vi "CloseSession.vi"   [LabVIEW 2023]
uses:
  Open_device_2018.llb/Select_Instr.ctl
types:
  T1 = typedef "Select_Instr.ctl" = string
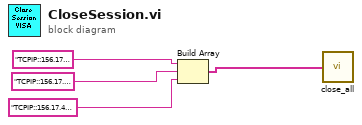
[diagram p0: block diagram]
diagram:
  n1 = Build Array(T1 "TCPIP::156.17.45.35::inst18::INSTR" ("Select_Instrument"), T1 "TCPIP::156.17.45.35::inst19::INSTR" ("Select_Instrument"), T1 "TCPIP::156.17.45.35::inst21::INSTR" ("Select_Instrument")) -> (w1:T1[])
  n2 = call "close_all.vi"("OpenRes"=w1) -> ()  [unwired: 1 out]
